vi "HandShaking.vi"(6 "Elapsed Time":u32, 8 "error in (no error)":errorcluster, 10 "Event Sources":T1, 11 "PostUUT in":refnum<class "PostUUT.lvclass">) -> (0 "error out":errorcluster, 3 "PostUUT out":refnum<class "PostUUT.lvclass">)   [LabVIEW 2021, in "PostUUT.lvclass"]
uses:
  PostUUT.lvclass
  PostUUT.lvclass/PostUUT.ctl
  OPC UA/OPC UA.lvclass
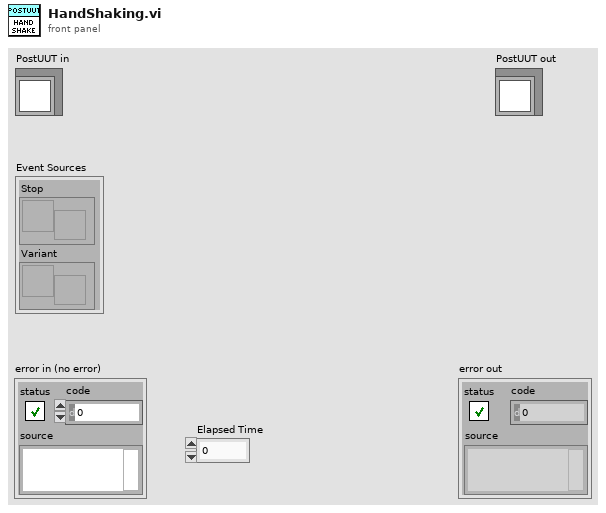
[diagram p1: front panel]
types:
  T1 = cluster{"Stop":refnum<user-event>, "Variant":refnum<user-event>}
  T2 = typedef "PostUUT.lvclass/Rx PostUUT.ctl" = cluster{"ResultsAck":bool, "Reset":bool, "Stop":bool, "FaultCode":u32}
  T3 = typedef "PostUUT.lvclass/Tx PostUUT.ctl" = cluster{"ResultsReady":bool, "Results":i32, "ElapsedTime":i32, "TimeCompleted":i32[], "Fault":bool, "Timeout":bool}
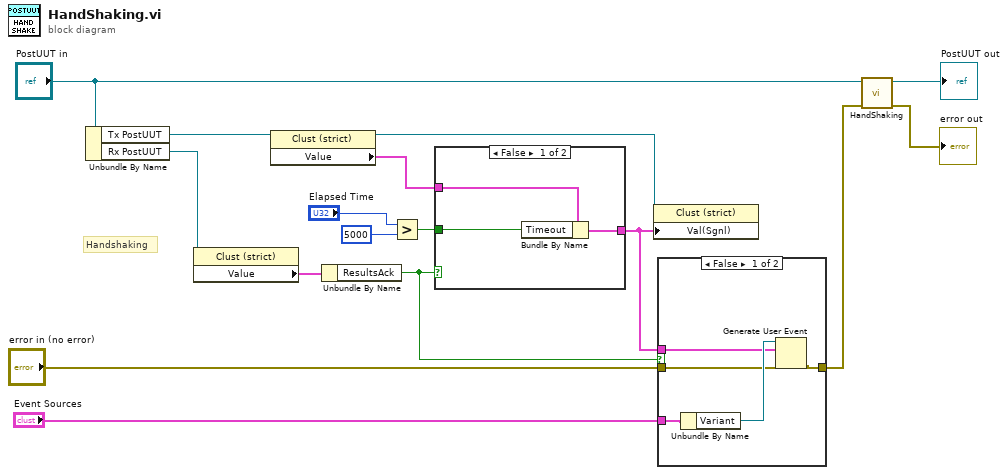
[diagram p0: block diagram]
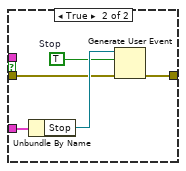
[diagram p2: hidden frame]
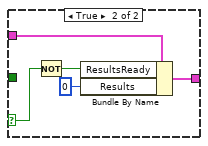
[diagram p3: hidden frame]
diagram:
  # "Handshaking"
  n1 = Unbundle By Name("PostUUT in") -> ("Tx PostUUT"=w11:refnum<vi>, "Rx PostUUT"=w12:refnum<vi>)
  n2 = property class="Clust (strict)"(reference=w12) -> ("Value"=w13:T2)  [unwired: 1 in, 2 out]
  n3 = property class="Clust (strict)"(reference=w11) -> (reference out=w14:refnum<vi>, "Value"=w15:T3)  [unwired: 1 in, 1 out]
  n4 = Unbundle By Name(w13) -> ("ResultsAck"=w4:bool)
  n5 = Greater?(x="Elapsed Time", y=u32 5000) -> (0:w7:bool)
  n6 = case shown="False" w4 {
    selector: w4 -> [_ w21]
    tunnel: w15 -> [w19 w23]
    tunnel: [w18 w22] -> w3
    tunnel: w7 -> [w17 _]
    frame False {
      n7 = Bundle By Name(cluster=w19, "Timeout"=w17) -> (w18:T3)
    }
    frame True {
      n8 = Not(x=w21) -> (.not. x?=w20:bool)
      n9 = Bundle By Name(cluster=w23, "ResultsReady"=w20, "Results"=0) -> (w22:T3)
    }
  }
  n10 = property class="Clust (strict)"(reference=w14, "Val(Sgnl)"=w3) -> ()  [unwired: 1 in, 2 out]
  n11 = case shown="False" w4 {
    tunnel: "Event Sources" -> [w29 w34]
    tunnel: w3 -> [w27 _]
    tunnel: "error in (no error)" -> [w26 w31]
    tunnel: [w25 w30] -> w1
    frame False {
      n12 = Unbundle By Name(w29) -> ("Variant"=w28:refnum<user-event>)
      n13 = Generate User Event(user event=w28, event data cluster=w27, error in=w26) -> (error out=w25:errorcluster)  [unwired: 1 in, 1 out]
    }
    frame True {
      w32 = TRUE  # Stop
      n14 = Unbundle By Name(w34) -> ("Stop"=w33:refnum<user-event>)
      n15 = Generate User Event(user event=w33, event data cluster=w32, error in=w31) -> (error out=w30:errorcluster)  [unwired: 1 in, 1 out]
    }
  }
  n16 = call-parent "HandShaking.vi"("error in (no error)"=w1, "OPC UA in"="PostUUT in") -> ("error out"=→"error out":errorcluster, "OPC UA out"=→"PostUUT out":refnum<class "PostUUT.lvclass">)  [unwired: 8 in]
